vi "Map_Update_Map_with_Forget_factor.vi"(8 "error in (no error)":errorcluster, 11 "Map in":dbl[][](array[numeric])) -> (0 "error out":errorcluster, 3 "Map out":dbl[][](array[numeric]))   [LabVIEW 2017]
uses:
  Simulator_SupportedVIs/GBL/GBL_variables.vi
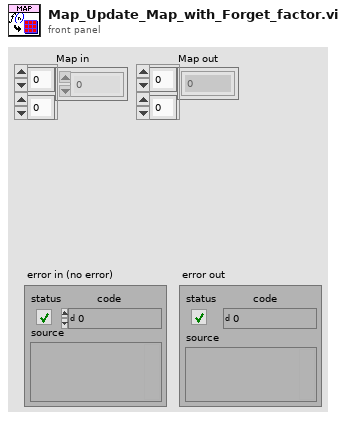
[diagram p1: front panel]
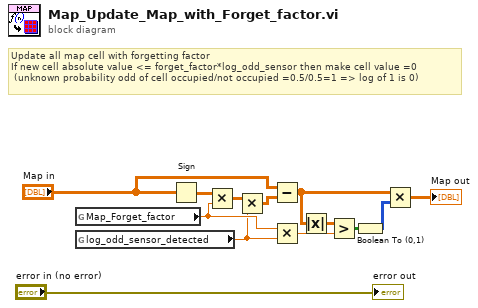
[diagram p0: block diagram]
diagram:
  # "Update all map cell with forgetting factor\nIf new cell absolute value <= forget_factor*log_odd_sensor then make cell value =0\n (unknown probability odd of cell occupied/not occupied =0.5/0.5=1 => log of 1 is 0)"
  n1 = global read "GBL_variables.vi" "Map_Forget_factor"() -> (w8:dbl)
  n2 = global read "GBL_variables.vi" "log_odd_sensor_detected"() -> (w7:dbl)
  n3 = Sign(1:"Map in") -> (0:w3:dbl[][])
  n4 = Multiply(x=w3, y=w8) -> (x*y=w4:dbl[][])
  n5 = Multiply(x=w4, y=w7) -> (x*y=w5:dbl[][])
  n6 = Subtract(x="Map in", y=w5) -> (x-y=w12:dbl[][])
  n7 = Multiply(x=w8, y=w7) -> (x*y=w10:dbl)
  n8 = Absolute Value(x=w12) -> (abs(x)=w9:dbl[][])
  n9 = Greater?(x=w9, y=w10) -> (0:w11:bool[][])
  n10 = Boolean To (0,1)(Boolean=w11) -> (0, 1=w13:i16[][])
  n11 = Multiply(x=w12, y=w13) -> (x*y=→"Map out":dbl[][])
  "error out" <- "error in (no error)"
